vi "GPS - Get Reading_SubVI.vi"(8 "error in (no error) 2":errorcluster) -> (0 "error out":errorcluster, 1 "Longitude W (deg)":dbl, 2 "Latitude N (deg)":dbl, 3 "GNRMC String Array":string[](array[string]), 5 "VISA resource name out":refnum<visa-resource-name>)   [LabVIEW 2021]
uses:
  <vilib>/myRIO/Instrument Drivers/Onboard IO/UART/typedef/VISA Configuration.ctl
  <vilib>/Instr/_visa.llb/VISA Configure Serial Port (Instr).vi
  <vilib>/myRIO/Instrument Drivers/Onboard IO/UART/UART.lvlib
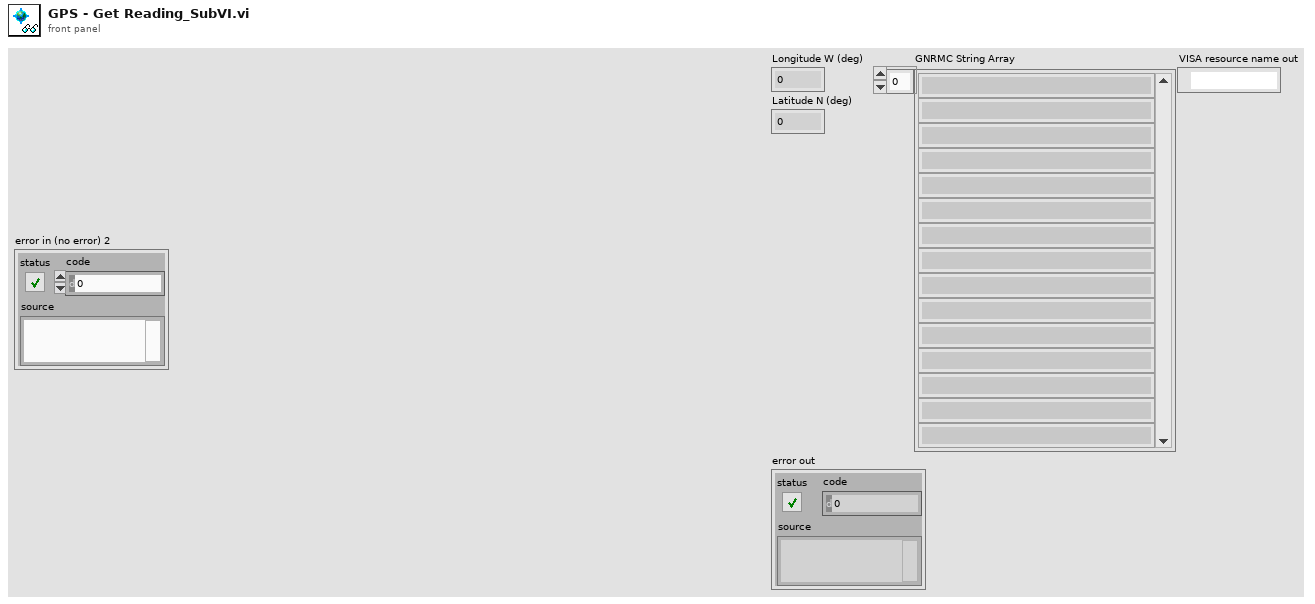
[diagram p1: front panel]
types:
  T1 = typedef "UART.lvlib/VISA Configuration.ctl" = cluster{"baud rate (9600)":u32, "data bits (8)":u16, "parity (0:none)":enum16{"None", "Odd", "Even", "Mark", "Space"}, "stop bits (10: 1 bit)":u16, "flow control (0:none)":u16, "termination char\n(0xA = '\\n' = LF) ":u8, "Enable Termination\nChar (T)":bool, "timeout (10sec)":u32}
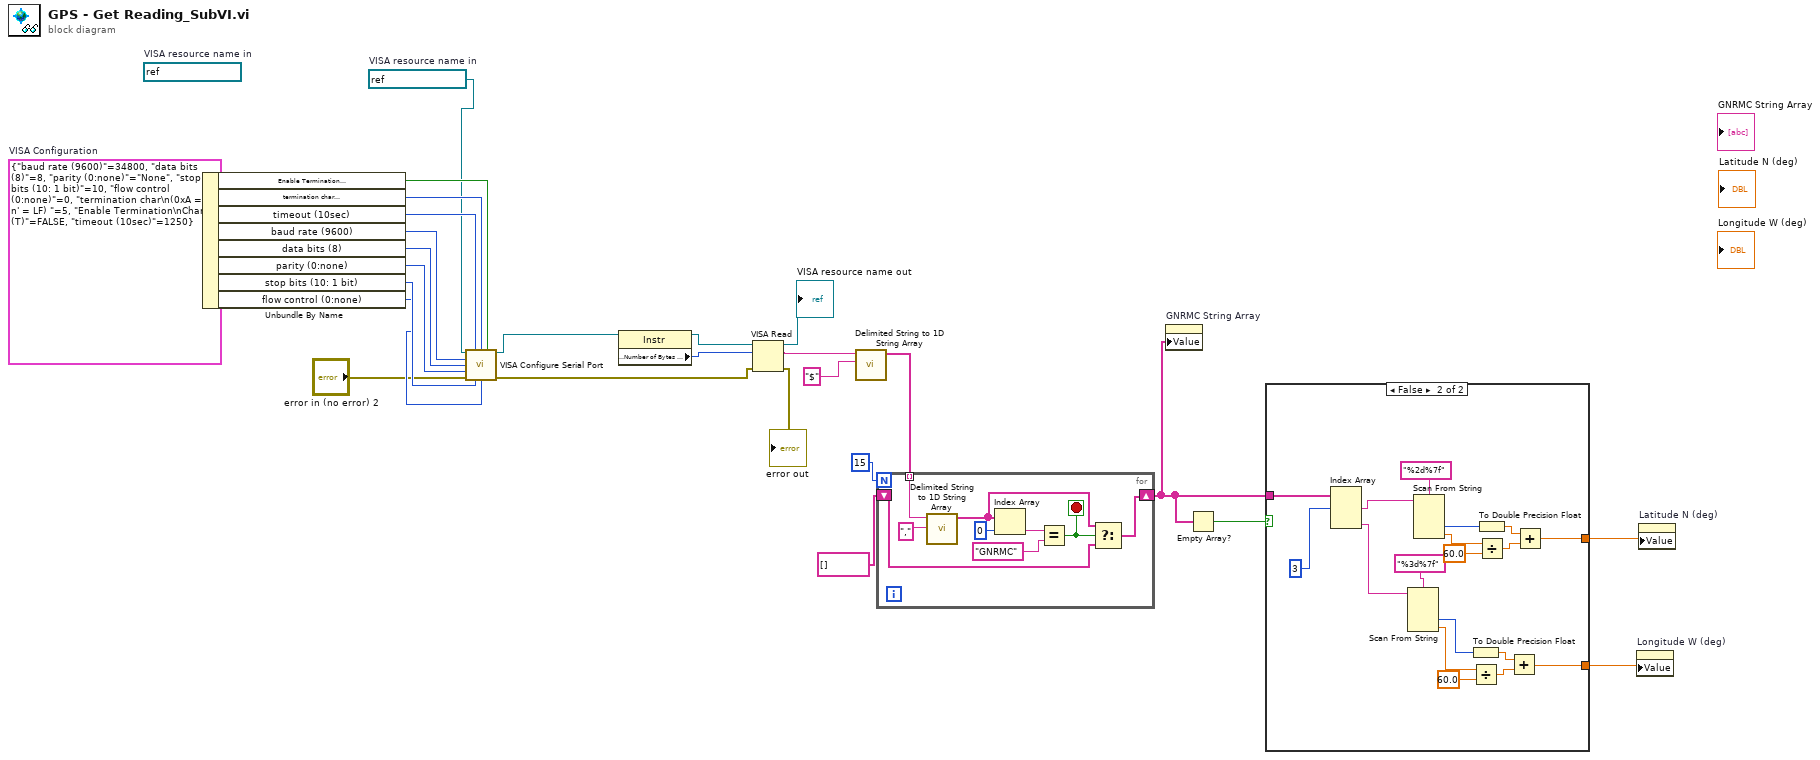
[diagram p0: block diagram]
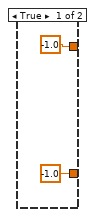
[diagram p2: hidden frame]
diagram:
  w4 = refnum<visa-resource-name> "ASRL1::INSTR"  # VISA resource name in
  (unwired) refnum<visa-resource-name> "ASRL2::INSTR"  # VISA resource name in
  w5 = T1 {"baud rate (9600)"=34800, "data bits (8)"=8, "parity (0:none)"=enum."None", "stop bits (10: 1 bit)"=10, "flow control (0:none)"=0, "termination char\n(0xA = '\\n' = LF) "=5, "Enable Termination\nChar (T)"=FALSE, "timeout (10sec)"=1250}  # VISA Configuration
  n1 = Unbundle By Name(w5) -> ("Enable Termination\nChar (T)"=w7:bool, "termination char\n(0xA = '\\n' = LF)"=w8:u8, "timeout (10sec)"=w9:u32, "baud rate (9600)"=w14:u32, "data bits (8)"=w13:u16, "parity (0:none)"=w12:enum16{"None", "Odd", "Even", "Mark", "Space"}, "stop bits (10: 1 bit)"=w11:u16, "flow control (0:none)"=w10:u16)
  n2 = call-poly "VISA Configure Serial Port"("VISA resource name"=w4, "timeout (10sec)"=w9, "termination char\n(0xA = '\\n' = LF)"=w8, "Enable Termination\nChar (T)"=w7, "baud rate (9600)"=w14, "data bits (8)"=w13, "parity (0:none)"=w12, "error in (no error)"="error in (no error) 2", "stop bits (10: 1 bit)"=w11, "flow control (0:none)"=w10) -> ("VISA resource name out"=w3:refnum<visa-resource-name>, "error out"=w2:errorcluster)  [unwired: 4 in]
  n3 = property class="Instr"(reference=w3) -> (reference out=w16:refnum<visa-resource-name>, "Serial Settings:Number of Bytes at Serial Port"=w15:u32)  [unwired: 1 in, 1 out]
  n4 = VISA Read(VISA resource name=w16, byte count=w15, error in (no error)=w2) -> (VISA resource name out=→"VISA resource name out":refnum<visa-resource-name>, read buffer=w21:string, error out=→"error out":errorcluster)  [unwired: 1 out]
  n5 = call <vilib>:"Delimited String to 1D String Array.vi"("delimiter"="$" ("delimiter (Tab)"), "delimited string"=w21) -> ("string array"=w26:string[])  [unwired: 9 in]
  n6 = for {
    N: 15 -> [_]
    tunnel: w26 -> [w35] mode=indexing
    shift-right: [w27] -> w19
    shift-left: string[] [] -> [w28]
    stop <- w30 stop-if-true
    n7 = call <vilib>:"Delimited String to 1D String Array.vi"("delimiter"=",", "delimited string"=w35) -> ("string array"=w29:string[])  [unwired: 9 in]
    n8 = Index Array(array=w29, index=0) -> (element=w33:string)
    n9 = Equal?(x=w33, y="GNRMC" ("element")) -> (x = y?=w30:bool)
    n10 = Select(t=w29, s=w30, f=w28) -> (s? t:f=w27:string[])
  }
  n11 = property on="GNRMC String Array" class="Arr (strict)"("Value"=w19) -> ()  [unwired: 2 in, 2 out]
  n12 = Empty Array?(array=w19) -> (empty?=w22:bool)
  n13 = case shown="False" w22 {
    tunnel: [-1.0 w54] -> w17
    tunnel: [-1.0 w53] -> w18
    tunnel: w19 -> [_ w38]
    frame True {
    }
    frame False {
      n14 = Index Array(array=w38, index #1=3 ("index")) -> (element #1=w39:string, element #3=w52:string)  [unwired: 2 in, 1 out]
      n15 = Scan From String(format string="%3d%7f", input string=w52) -> (output 1=w49:i32, output 2=w47:dbl)  [unwired: 4 in, 3 out]
      n16 = Scan From String(format string="%2d%7f", input string=w39) -> (output 1=w43:i32, output 2=w41:dbl)  [unwired: 4 in, 3 out]
      n17 = To Double Precision Float(number=w49) -> (double precision float=w50:dbl)
      n18 = Divide(x=w47, y=60.0) -> (x/y=w51:dbl)
      n19 = To Double Precision Float(number=w43) -> (double precision float=w44:dbl)
      n20 = Divide(x=w41, y=60.0) -> (x/y=w45:dbl)
      n21 = Add(x=w50, y=w51) -> (x+y=w54:dbl)
      n22 = Add(x=w44, y=w45) -> (x+y=w53:dbl)
    }
  }
  n23 = property on="Longitude W (deg)" class="DigNum (strict)"("Value"=w17) -> ()  [unwired: 2 in, 2 out]
  n24 = property on="Latitude N (deg)" class="DigNum (strict)"("Value"=w18) -> ()  [unwired: 2 in, 2 out]
